vi "题目5.vi"() -> ()   [LabVIEW 2017]
panel:
  in  "停止":bool
  out "恭喜":bool
  out "通过":bool
  out "警告":bool
  in  "数值":i32
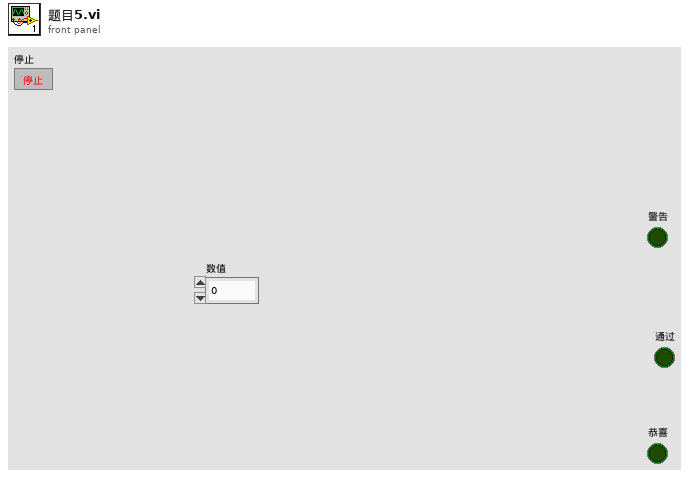
[diagram p1: front panel]
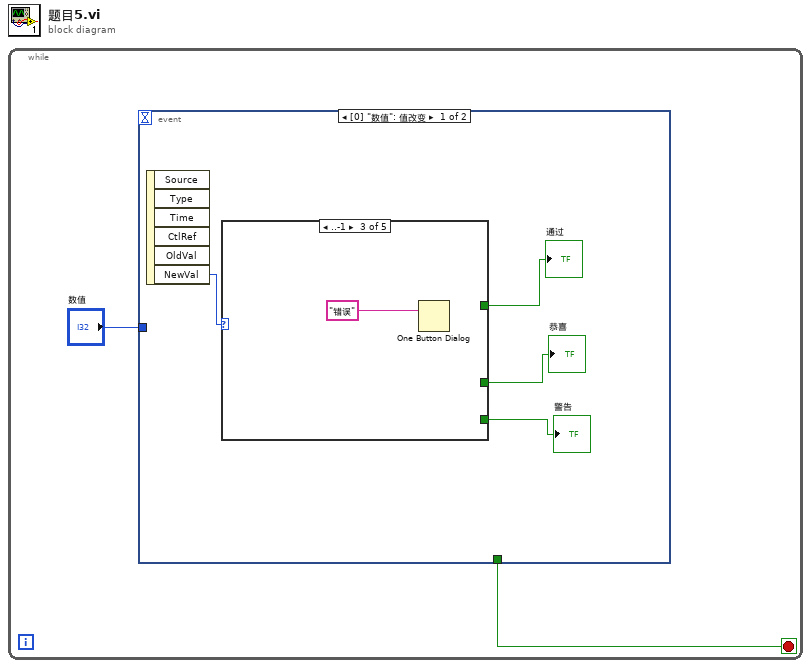
[diagram p0: block diagram]
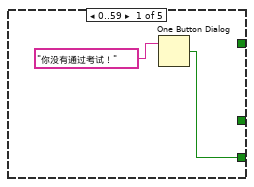
[diagram p2: hidden frame]
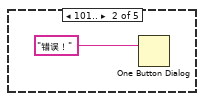
[diagram p3: hidden frame]
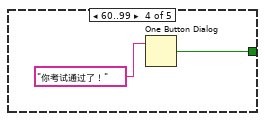
[diagram p4: hidden frame]
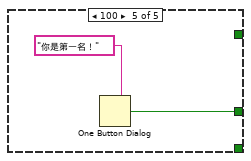
[diagram p5: hidden frame]
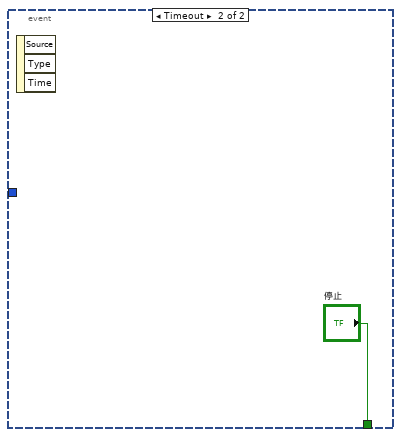
[diagram p6: hidden frame]
diagram:
  n1 = while {
    stop <- w1 stop-if-true
    n2 = event shown="[0] \"数值\": 值改变" {
      selector: _ -> [_ _]
      dyn-events: _ -> [_ _]
      timeout: _ -> [_ _]
      tunnel: "数值" -> [_ _]
      tunnel: [_ "停止"] -> w1
      event "数值": Value Change {
        n3 = event-data() -> ("NewVal"=w3:i32)  [unwired: 1 in, 5 out]
        n4 = case shown="..-1" w3 {
          tunnel: [_ _ _ w11 _] -> w6
          tunnel: [_ _ _ _ w13] -> w5
          tunnel: [w7 _ _ _ _] -> w4
          frame 0..59 {
            n5 = One Button Dialog(message="你没有通过考试！") -> (true=w7:bool)  [unwired: 1 in]
          }
          frame 101.. {
            n6 = One Button Dialog(message="错误！") -> ()  [unwired: 1 in, 1 out]
          }
          frame ..-1 {
            n7 = One Button Dialog(message="错误") -> ()  [unwired: 1 in, 1 out]
          }
          frame 60..99 {
            n8 = One Button Dialog(message="你考试通过了！") -> (true=w11:bool)  [unwired: 1 in]
          }
          frame 100 {
            n9 = One Button Dialog(message="你是第一名！") -> (true=w13:bool)  [unwired: 1 in]
          }
        }
        "通过" <- w6
        "恭喜" <- w5
        "警告" <- w4
      }
      event Timeout {
        n10 = event-data() -> ()  [unwired: 1 in, 3 out]
      }
    }
  }
